vi "YKMW100 Computation Control.vi"(0 "VISA session":refnum<visa-resource-name>="MW100", 5 "Mode":T1(ring), 11 "error in (no error)":errorcluster) -> (4 "dup VISA session":refnum<visa-resource-name>="MW100", 15 "error out":errorcluster)   [LabVIEW 2016]
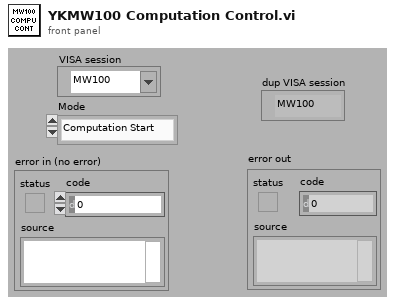
[diagram p1: front panel]
types:
  T1 = enum16{"Computation Start", "Computation stop", "Reset Computation", "Clear Computation"}
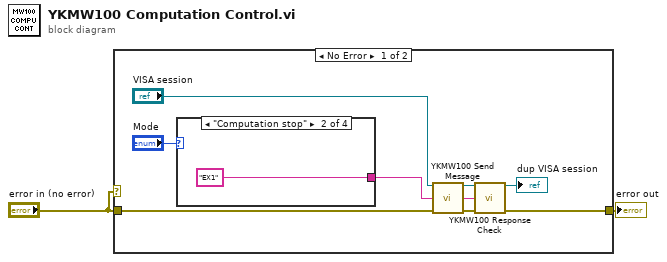
[diagram p0: block diagram]
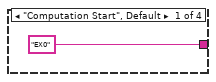
[diagram p2: hidden frame]
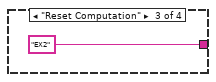
[diagram p3: hidden frame]
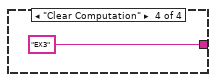
[diagram p4: hidden frame]
diagram:
  n1 = case shown="No Error" "error in (no error)" {
    tunnel: "error in (no error)" -> [w10 w16]
    tunnel: [w6 w16] -> w2
    frame No Error {
      n2 = case shown="\"Computation stop\"" "Mode" {
        tunnel: ["EX0" ("Send Message (\"\")") "EX1" ("Send Message (\"\")") "EX2" ("Send Message (\"\")") "EX3" ("Send Message (\"\")")] -> w9
        frame "Computation Start", Default {
        }
        frame "Computation stop" {
        }
        frame "Reset Computation" {
        }
        frame "Clear Computation" {
        }
      }
      n3 = call "YKMW100 Send Message.vi"("VISA session"="VISA session", "Send Message (\"\")"=w9, "error in (no error)"=w10) -> ("dup VISA session"=w3:refnum<visa-resource-name>, "Read Buffer"=w4:string, "error out"=w5:errorcluster)  [unwired: 10 in]
      n4 = call "YKMW100 Response Check.vi"("VISA session"=w3, "Message In (\"\")"=w4, "error in (no error)"=w5) -> ("dup VISA session"=→"dup VISA session":refnum<visa-resource-name>, "error out"=w6:errorcluster)  [unwired: 8 in, 3 out]
    }
    frame Error {
    }
  }
  "error out" <- w2
